vi "WILT Parse Agilent Channel List.vi"(8 "Error In":errorcluster, 11 "Array":T1[](array[typedef])) -> (0 "Error Out":errorcluster, 1 "Configure Scan List":string, 2 "Resistance":string, 3 "Voltage":string, 4 "Number of Read Channels":i32, 5 "Current":string, 6 "Channel List":string, 7 "Temperature":string)   [LabVIEW 2016]
uses:
  Type Definitions/WILT Agilent Channel Definition.ctl
  <vilib>/Utility/error.llb/whitespace.ctl
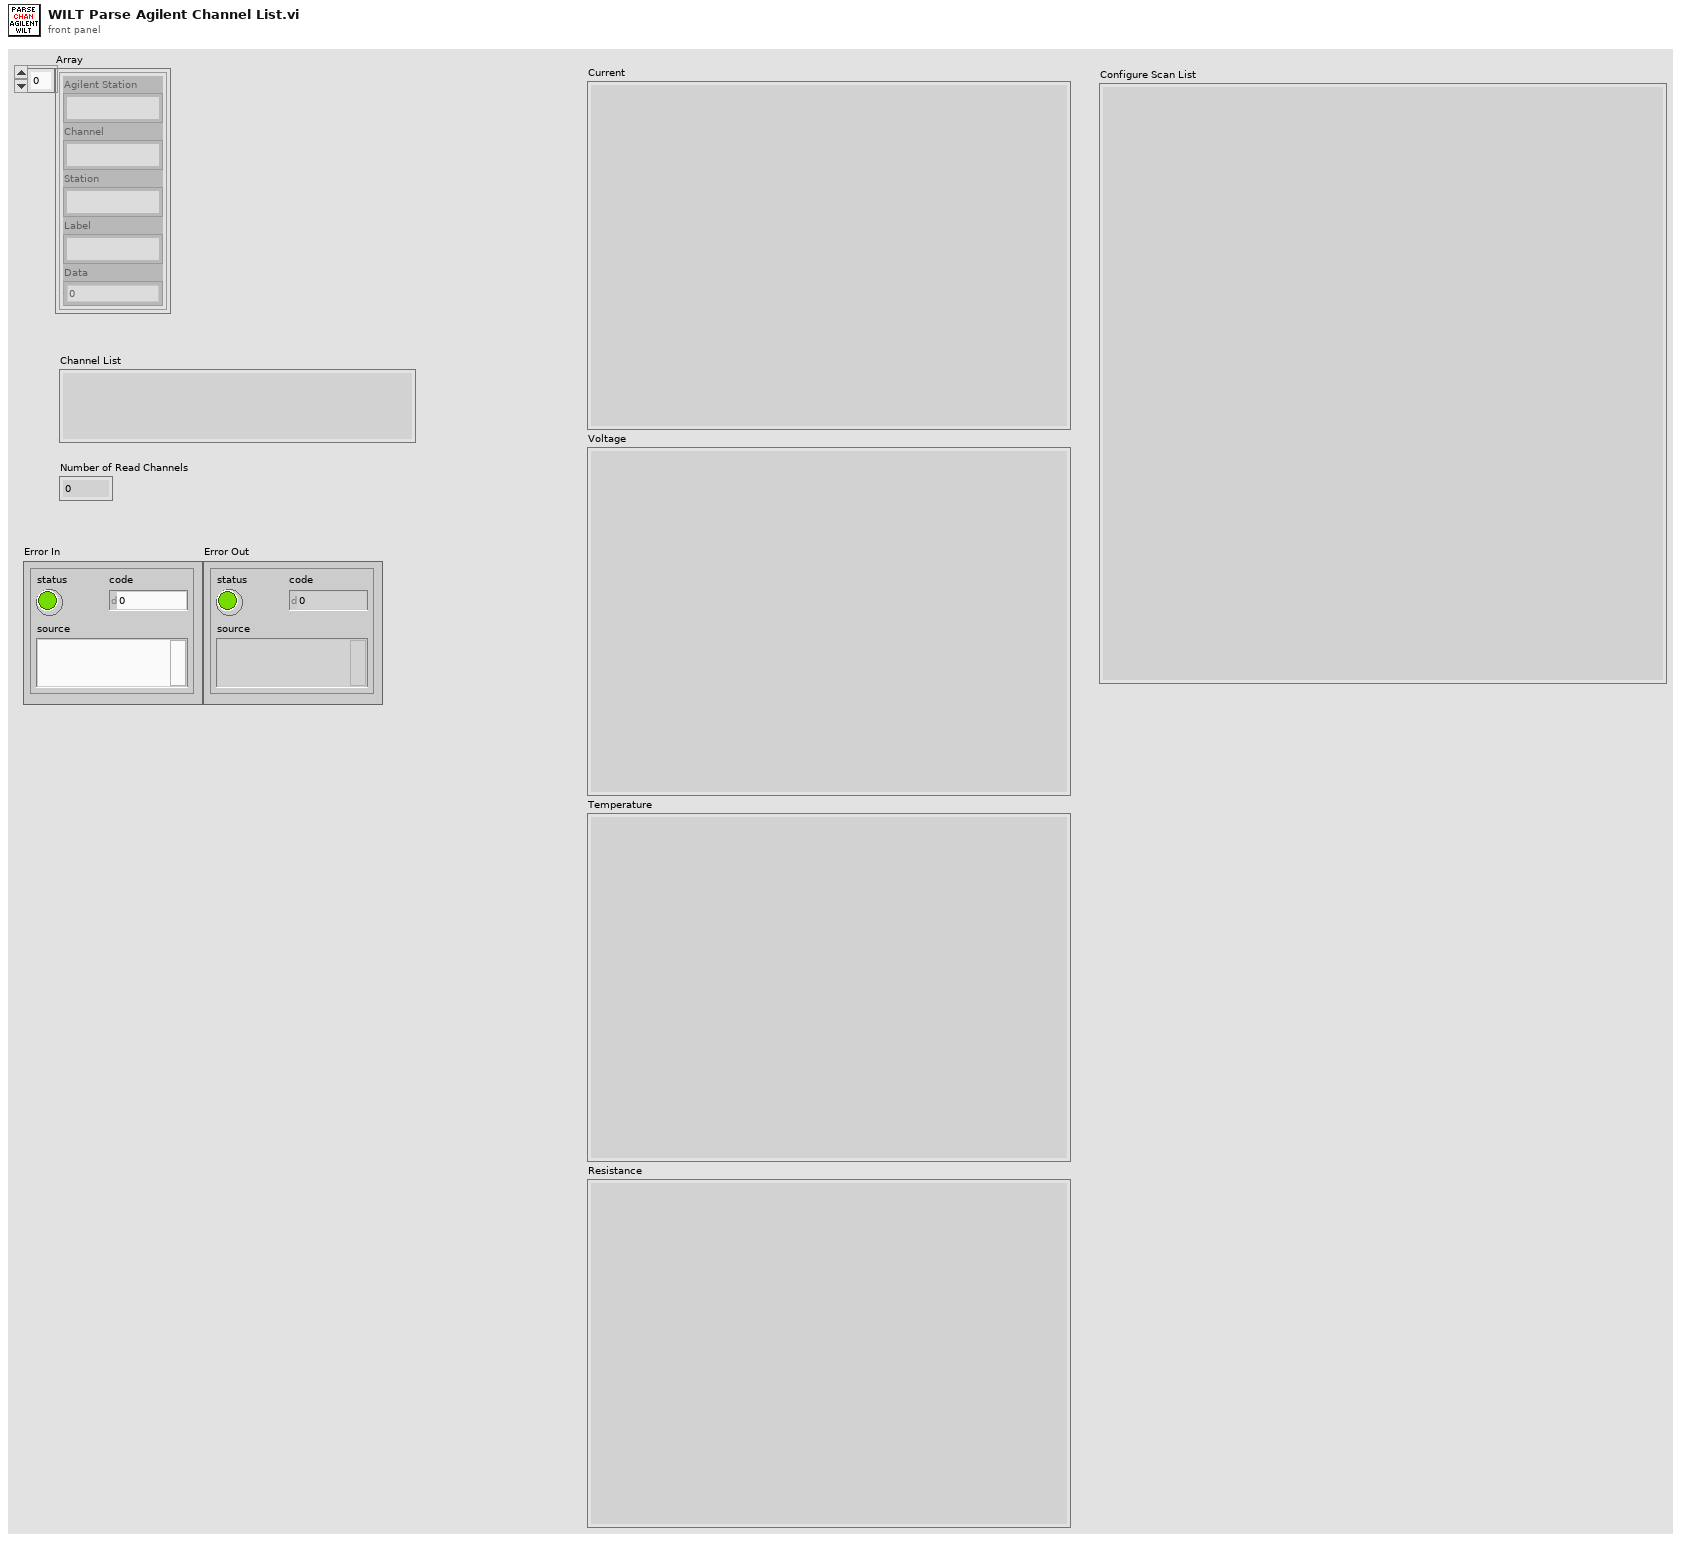
[diagram p1: front panel]
types:
  T1 = typedef "WILT Agilent Channel Definition.ctl" = cluster{"Channel":string, "Station":string, "Label":string, "Agilent Station":string, "Data":dbl}
  T2 = typedef "whitespace.ctl" = u16
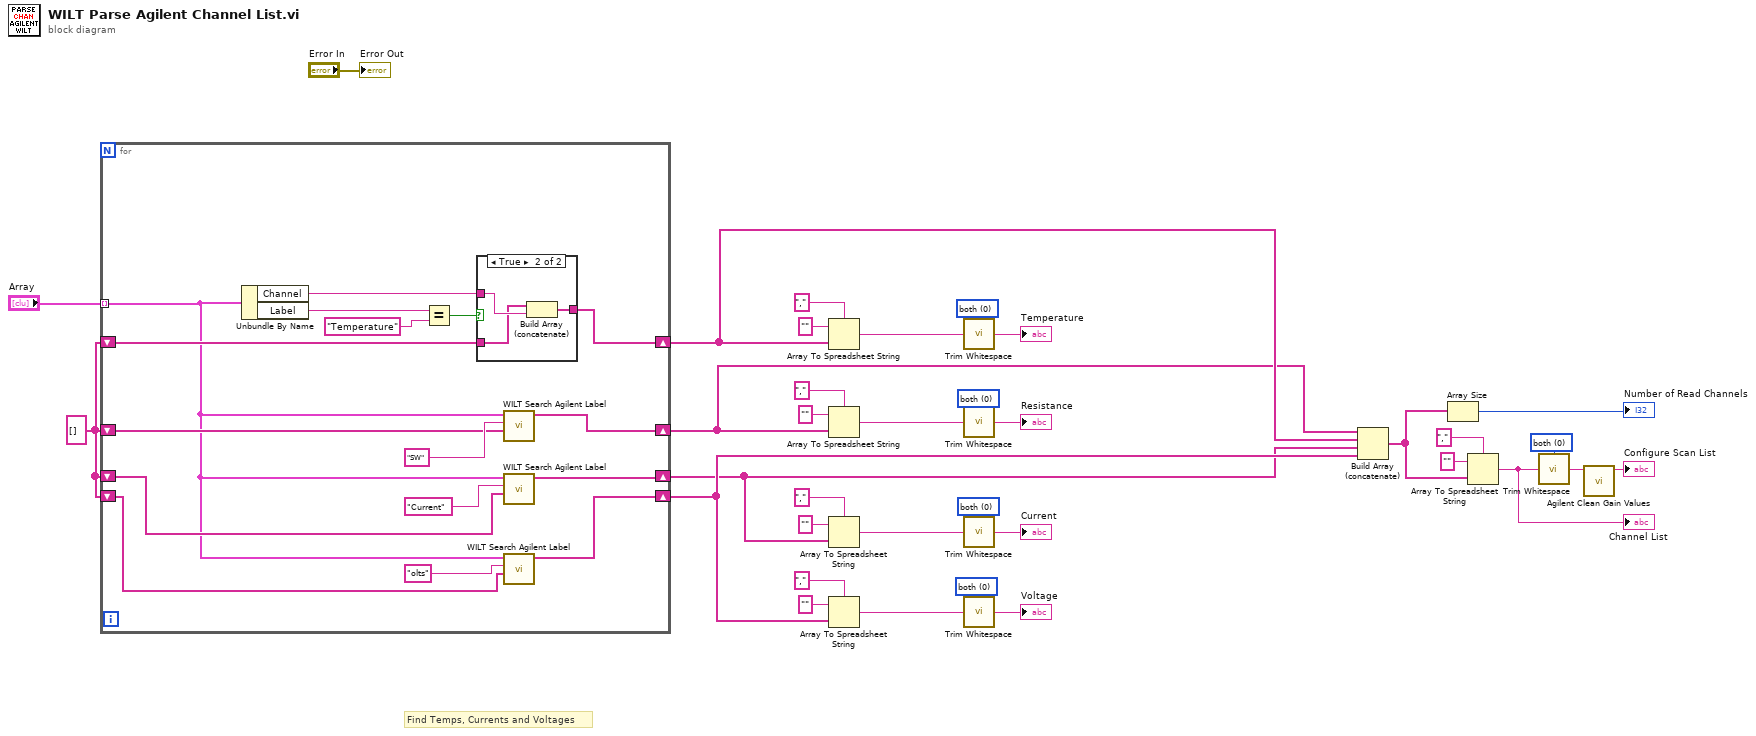
[diagram p0: block diagram]
diagram:
  w3 = T2 0 items=["both", "start of string", "end of string"] ("location (both)")
  w4 = T2 0 items=["both", "start of string", "end of string"] ("location (both)")
  w5 = T2 0 items=["both", "start of string", "end of string"] ("location (both)")
  w6 = T2 0 items=["both", "start of string", "end of string"] ("location (both)")
  w7 = T2 0 items=["both", "start of string", "end of string"] ("location (both)")
  w16 = string[] []
  # "Find Temps, Currents and Voltages"
  n1 = for {
    tunnel: "Array" -> [w39] mode=indexing
    shift-right: [w49] -> w34
    shift-left: w16 -> [w48]
    shift-right: [w40] -> w22
    shift-left: w16 -> [w41]
    shift-right: [w36] -> w23
    shift-left: w16 -> [w37]
    shift-right: [w46] -> w21
    shift-left: w16 -> [w45]
    n2 = Unbundle By Name(w39) -> ("Channel"=w44:string, "Label"=w43:string)
    n3 = Equal?(x=w43, y="Temperature") -> (x = y?=w50:bool)
    n4 = case shown="True" w50 {
      tunnel: w44 -> [_ w55]
      tunnel: [w52 w54] -> w49
      tunnel: w48 -> [w52 w53]
      frame False {
      }
      frame True {
        n5 = Build Array (concatenate)(w53, w55) -> (w54:string[])
      }
    }
    n6 = call "WILT Search Agilent Label.vi"("Array in"=w45, "Search For"="SW" ("regular expression"), "Agilent Channel Definition"=w39) -> ("Array out"=w46:string[])  [unwired: 7 in, 1 out]
    n7 = call "WILT Search Agilent Label.vi"("Array in"=w41, "Search For"="Current" ("regular expression"), "Agilent Channel Definition"=w39) -> ("Array out"=w40:string[])  [unwired: 7 in, 1 out]
    n8 = call "WILT Search Agilent Label.vi"("Array in"=w37, "Search For"="olts" ("regular expression"), "Agilent Channel Definition"=w39) -> ("Array out"=w36:string[])  [unwired: 7 in, 1 out]
  }
  n9 = Array To Spreadsheet String(delimiter (Tab)=",", array=w34, 3:"" ("format string")) -> (spreadsheet string=w26:string)
  n10 = Array To Spreadsheet String(delimiter (Tab)=",", array=w21, 3:"" ("format string")) -> (spreadsheet string=w35:string)
  n11 = Array To Spreadsheet String(delimiter (Tab)=",", array=w22, 3:"" ("format string")) -> (spreadsheet string=w28:string)
  n12 = Array To Spreadsheet String(delimiter (Tab)=",", array=w23, 3:"" ("format string")) -> (spreadsheet string=w32:string)
  n13 = call <vilib>:"Trim Whitespace.vi"("string"=w26, "location (both)"=w7) -> ("trimmed string"=→"Temperature":string)
  n14 = call <vilib>:"Trim Whitespace.vi"("string"=w35, "location (both)"=w6) -> ("trimmed string"=→"Resistance":string)
  n15 = call <vilib>:"Trim Whitespace.vi"("string"=w28, "location (both)"=w5) -> ("trimmed string"=→"Current":string)
  n16 = call <vilib>:"Trim Whitespace.vi"("string"=w32, "location (both)"=w4) -> ("trimmed string"=→"Voltage":string)
  n17 = Build Array (concatenate)(w21, w34, w22, w23) -> (w24:string[])
  n18 = Array Size(array=w24) -> (size(s)=→"Number of Read Channels":i32)
  n19 = Array To Spreadsheet String(delimiter (Tab)=",", array=w24, 3:"" ("format string")) -> (spreadsheet string=w30:string)
  "Channel List" <- w30
  n20 = call <vilib>:"Trim Whitespace.vi"("string"=w30, "location (both)"=w3) -> ("trimmed string"=w2:string)
  n21 = call "Agilent Clean Gain Values.vi"("Analog Channels-List"=w2) -> ("String"=→"Configure Scan List":string)  [unwired: 9 in, 1 out]
  "Error Out" <- "Error In"
